vi "set oscp staple file.vi"(8 "error in":errorcluster, 10 "ocsp staple file":path, 11 "lvlibretls configurable context in":refnum<class "lvlibretls configurable context.lvclass">) -> (0 "error out":errorcluster, 3 "lvlibretls configurable context out":refnum<class "lvlibretls configurable context.lvclass">)   [LabVIEW 2016, in "lvlibretls configurable context.lvclass"]
uses:
  lvlibretls configurable context.lvclass
  lvlibretls configurable context.lvclass/lvlibretls configurable context.ctl
  lv tls dll.lvlib
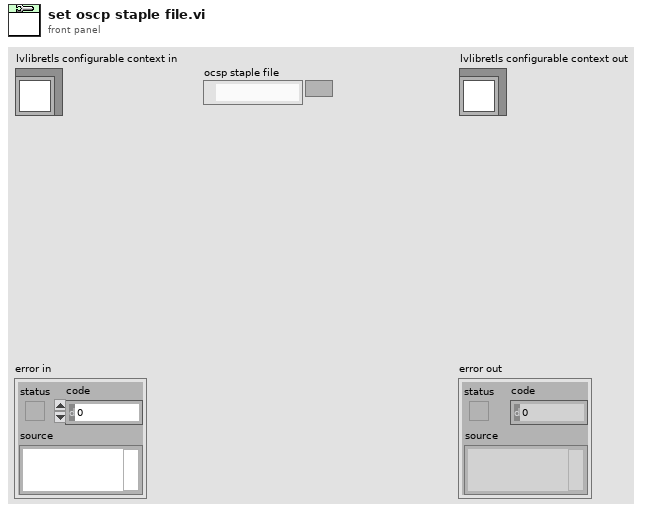
[diagram p1: front panel]
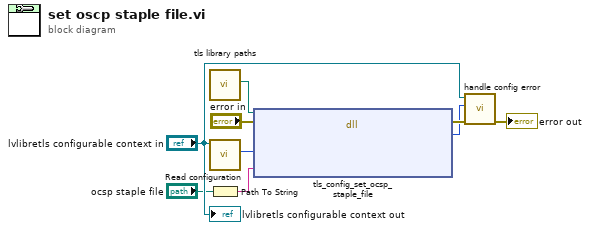
[diagram p0: block diagram]
diagram:
  n1 = call "tls library paths.vi"() -> ("libtls"=w9:path)  [unwired: 8 in, 3 out]
  n2 = call "Read configuration.vi"("lvlibretls configurable context in"="lvlibretls configurable context in") -> ("configuration"=w8:u64)  [unwired: 10 in]
  n3 = Path To String(path="ocsp staple file") -> (string=w1:string)
  n4 = dll-call lib="C:/Users/IEUser/Desktop/tlssimple/libtls-15.dll" fn="tls_config_set_ocsp_staple_file"(path in=w9, error in="error in", "config"=w8, "staplefile"=w1) -> (error out=w7:errorcluster, "return"=w6:i32)  [unwired: 3 in, 1 out]
  n5 = call "handle config error.vi"("error in"=w7, "return"=w6, "lvlibretls configurable context in"="lvlibretls configurable context in") -> ("error out"=→"error out":errorcluster)  [unwired: 8 in]
  "lvlibretls configurable context out" <- "lvlibretls configurable context in"
